vi "sendValue.vi"(8 "error in (no error)":errorcluster, 10 "data":variant, 11 "mainDoorState in":refnum<class "mainDoorState.lvclass">) -> (0 "error out":errorcluster, 2 "function return":i32, 3 "mainDoorState out":refnum<class "mainDoorState.lvclass">)   [LabVIEW 2016, in "SALLV_AtDome_Messaging.lvlib" / "mainDoorState.lvclass"]
uses:
  mainDoorState.lvclass
  ts_sallv_AtDome/DataTypes/logevent_mainDoorState.ctl
  ts_sallv_AtDome/SALLV_AtDome.lvlib
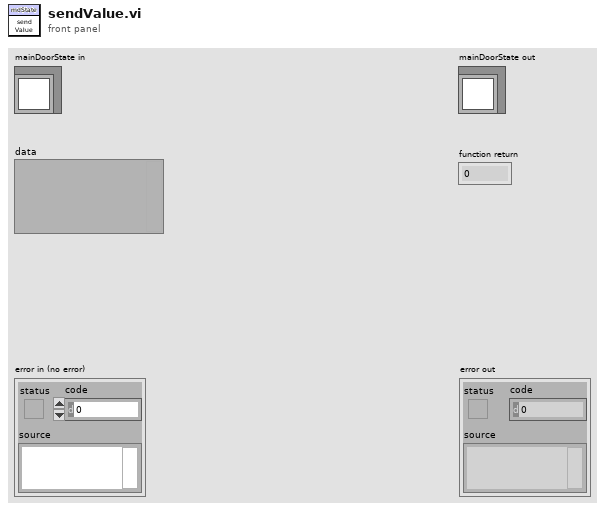
[diagram p1: front panel]
types:
  T1 = typedef "SALLV_AtDome.lvlib/logevent_mainDoorState.ctl" = cluster{"state":i32, "priority":i32}
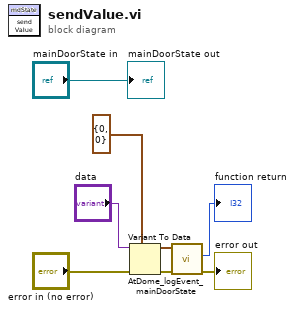
[diagram p0: block diagram]
diagram:
  n1 = Variant To Data(error in="error in (no error)", type=T1 {"state"=0, "priority"=0} ("data"), Variant="data") -> (data=w2:T1, error out=w5:errorcluster)
  n2 = call "AtDome_logEvent_mainDoorState.vi"("error in (no error)"=w5, "logevent_mainDoorState_Ctl"=w2) -> ("error out"=→"error out":errorcluster, "function return"=→"function return":i32)  [unwired: 7 in, 1 out]
  "mainDoorState out" <- "mainDoorState in"
